vi "Excel Driver.vi"(0 "Filename of Workbook":path, 2 "Operator":T1, 5 "WorkSheet Name":string="Sheet 1", 7 "Range String\n(Or Search String)":string, 9 "Cell Values INPUT":string[][](array[string]), 11 "error in (no error)":errorcluster) -> (4 "Cell Values OUT":string[][](array[string]), 6 "Returned Range":string[](array[string]), 15 "error out":errorcluster)   [LabVIEW 2019]
uses:
  Type Defs/Excel Driver Operator Type Def.ctl
panel:
  in  "Excel._Worksheet Typecast Reference":refnum<k7>
  in  "Excel._Application Starter Reference":refnum<k7>
  # "C:\\My Documents\\MyLabviewFiles\\MDMachines\\Machine list 12-02-2002a.xls"
  # "Machine List"
  # "\\\\Dlbm32221\\MachineFolders\\Machine list 12-02-2002a.xls"
  # "C:\\Documents and Settings\\tz92qf\\My Documents\\MyLabview\\MDMachines\\Machine list 12-02-2002a.xls"
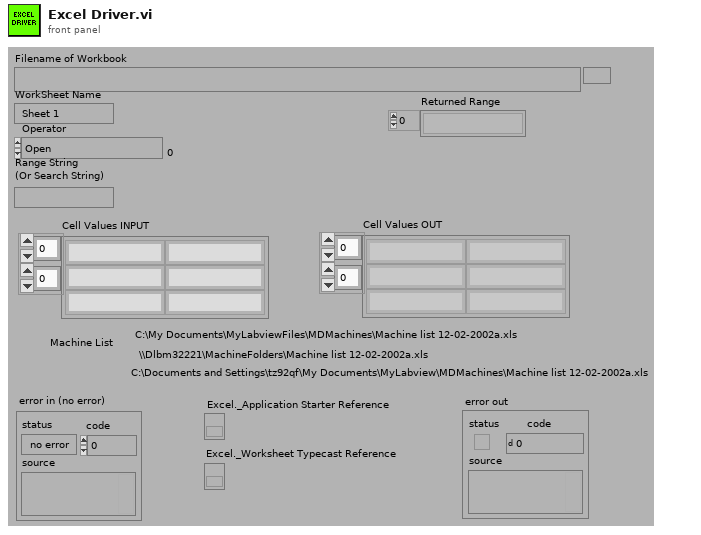
[diagram p1: front panel]
types:
  T1 = typedef "Excel Driver Operator Type Def.ctl" = enum16{"Open", "Close", "Search for String", "GetUsedRange", "Read Range", "Read Cell", "Set Range", "Set Cell"}
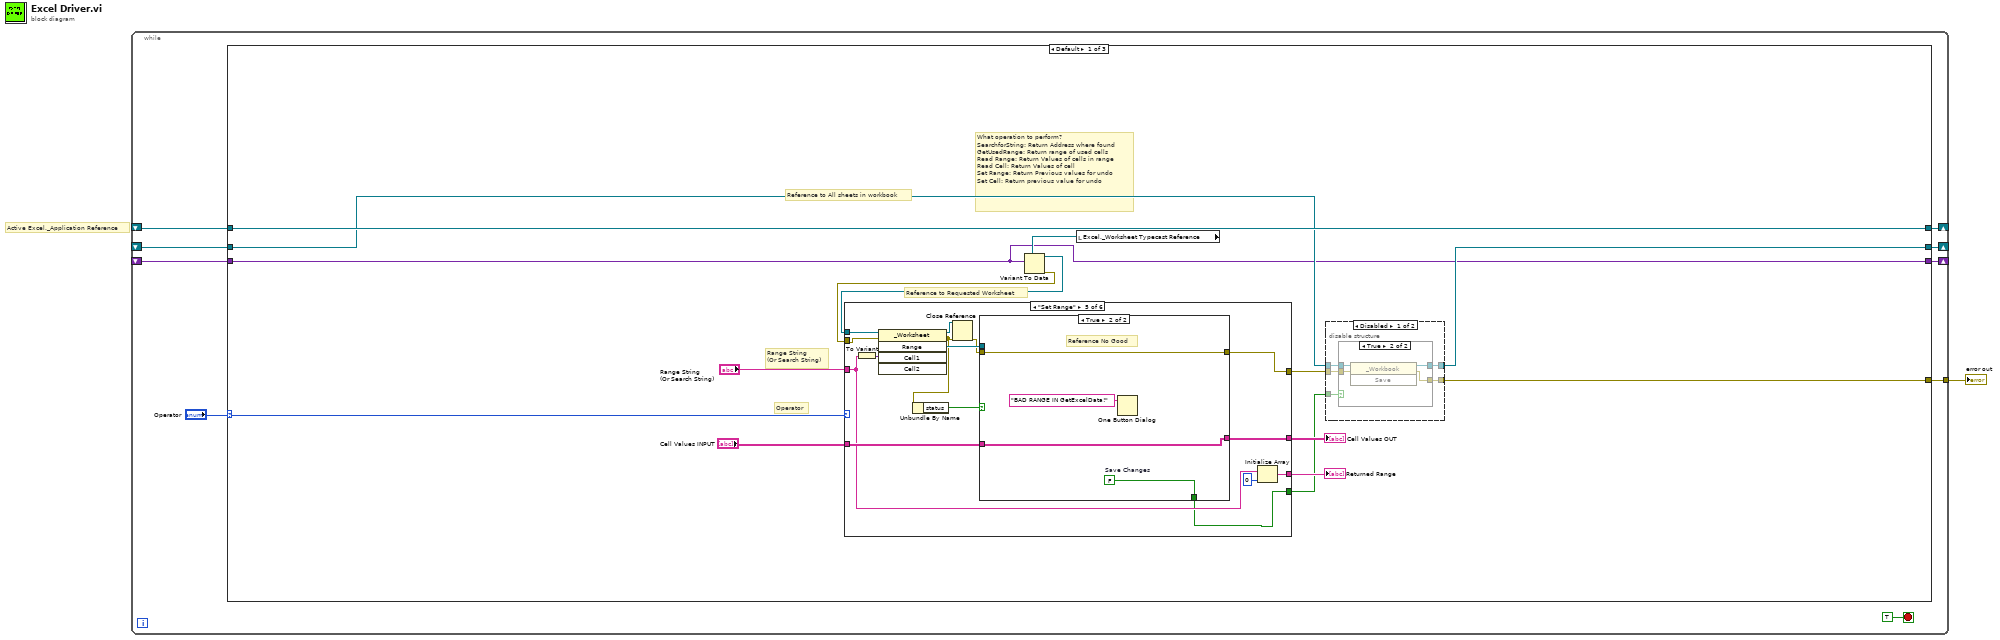
[diagram p0: block diagram]
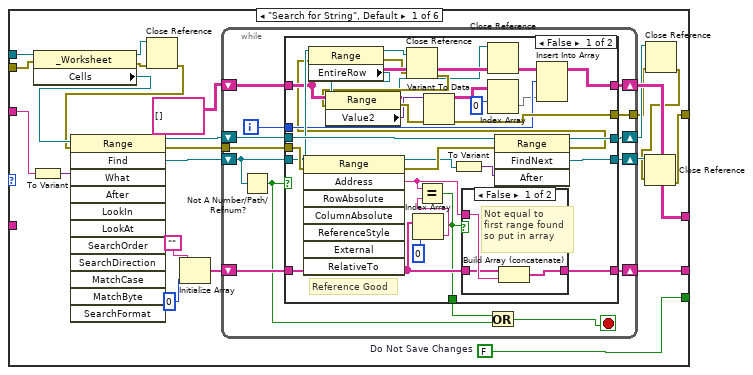
[diagram p4: hidden frame]
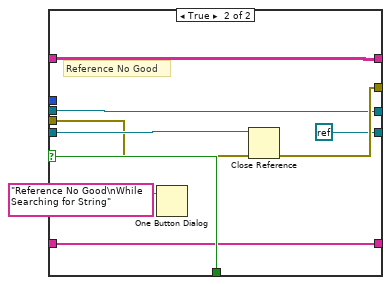
[diagram p6: hidden frame]
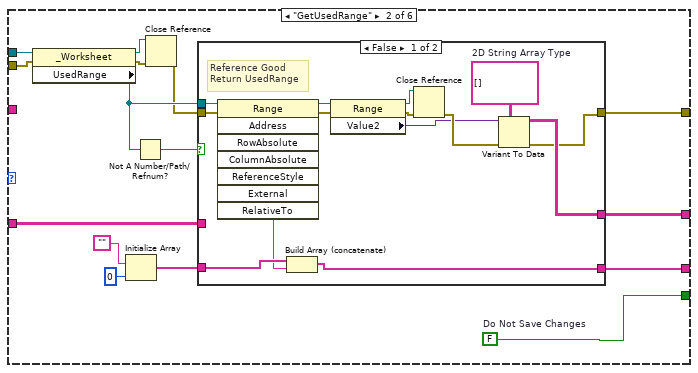
[diagram p7: hidden frame]
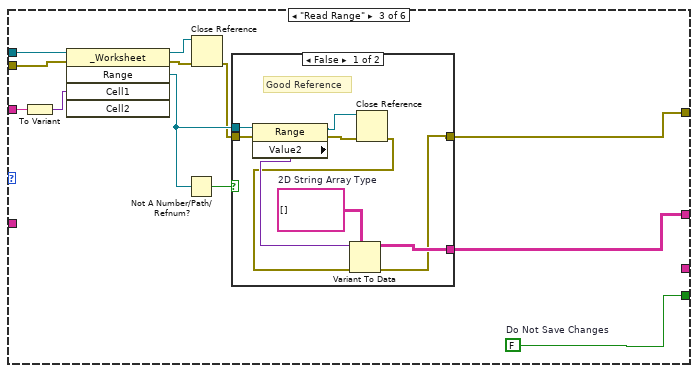
[diagram p9: hidden frame]
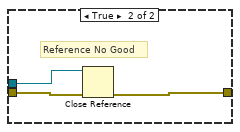
[diagram p10: hidden frame]
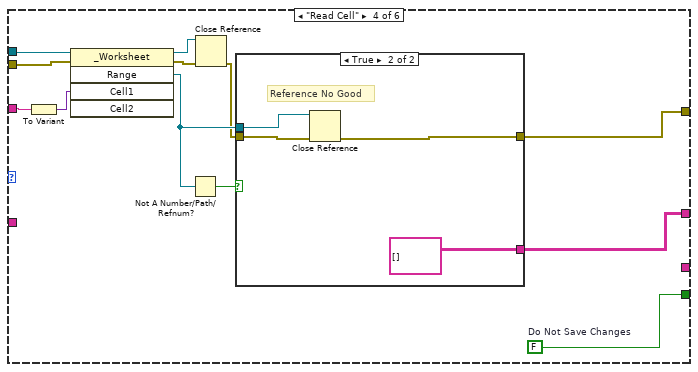
[diagram p11: hidden frame]
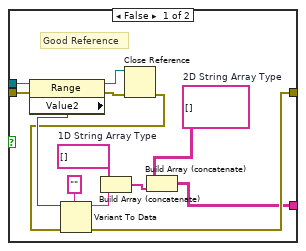
[diagram p12: hidden frame]
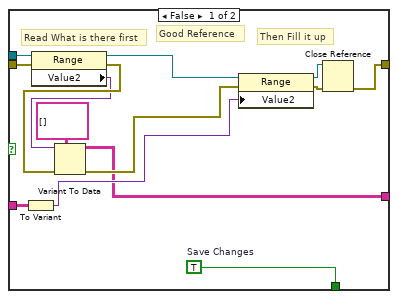
[diagram p13: hidden frame]
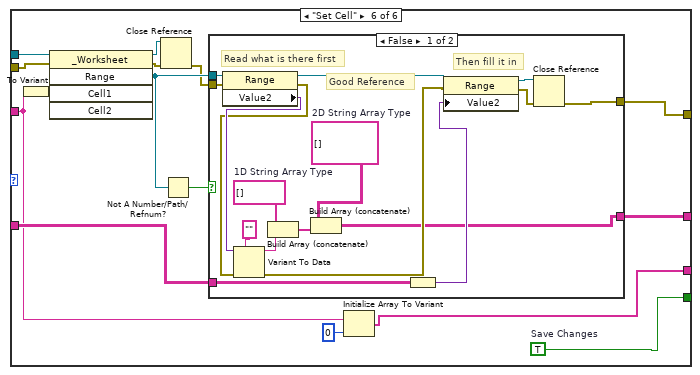
[diagram p14: hidden frame]
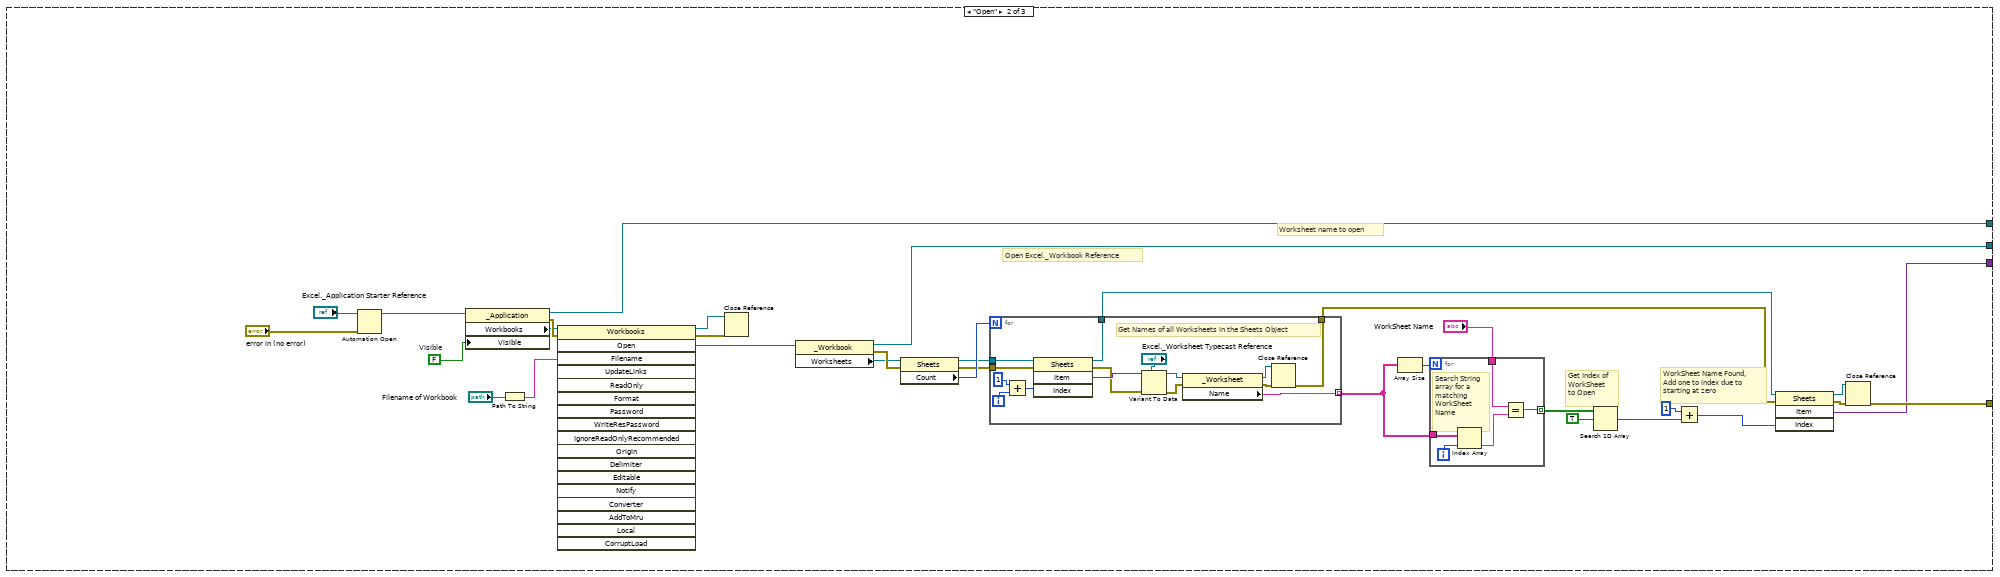
[diagram p16: hidden frame]
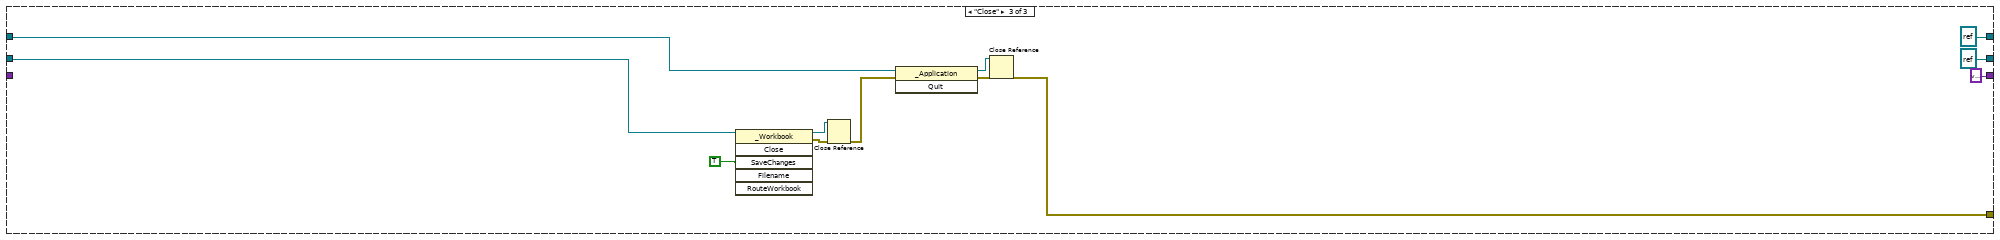
[diagram p17: hidden frame]
diagram:
  # "Active Excel._Application Reference"
  n1 = while {
    shift-right: [w10] -> _
    shift-left: _ -> [w9]
    tunnel: [w4] -> w1
    shift-right: [w6] -> _
    shift-left: _ -> [w5]
    shift-right: [w3] -> _
    shift-left: _ -> [w2]
    stop <- TRUE stop-if-true
    n2 = case shown="Default" "Operator" {
      selector: "Operator" -> [w24 _ _]
      tunnel: [w15 w280 refnum<k7> refnum ("Open")] -> w10
      tunnel: w9 -> [w16 _ w326]
      tunnel: [w19 w279 refnum<k7> refnum ("Excel._Application Starter Reference")] -> w6
      tunnel: w5 -> [w19 _ w327]
      tunnel: [w18 w271 w331] -> w4
      tunnel: [w11 w270 variant ("Item")] -> w3
      tunnel: w2 -> [w11 _ _]
      frame Default {
        # "Reference to Requested Worksheet"
        # "Range String\n(Or Search String)"
        # "Operator"
        # "Reference to All sheets in workbook"
        # "What operation to perform?\nSearchforString: Return Address where found\nGetUsedRange: Return range of used cells\nRead Range: Return Values of cells in range\nRead Cell: Return Values of cell\nSet Range: Return Previous values for undo\nSet Cell: Return previous value for undo"
        n3 = local read "Excel._Worksheet Typecast Reference"() -> (w12:refnum<k7>)
        n4 = Variant To Data(type=w12, Variant=w11) -> (data=w14:refnum<k7>, error out=w13:errorcluster)  [unwired: 1 in]
        n5 = case shown="\"Set Range\"" w24 {
          tunnel: w14 -> [w61 w130 w160 w177 w217 w245]
          tunnel: w13 -> [w60 w129 w161 w176 w216 w244]
          tunnel: "Range String\n(Or Search String)" -> [w59 _ w151 w175 w204 w239]
          tunnel: [w44 w126 w153 w178 w214 w241] -> w22
          tunnel: [w39 w118 w150 w174 w203 w236] -> w17
          tunnel: [w51 w122 _ _ w212 w237] -> w20
          tunnel: [w46 w120 w152 w179 w215 w240] -> w21
          tunnel: "Cell Values INPUT" -> [_ w119 _ _ w205 w242]
          frame "Search for String", Default {
            w39 = FALSE  # Do Not Save Changes
            n6 = To Variant(anything=w59) -> (Variant=w55:variant)
            n7 = property class="_Worksheet"(reference=w61, error in=w60) -> (reference out=w58:refnum<k7>, error out=w57:errorcluster, "Cells"=w56:refnum<k7>)
            n8 = Close Reference(reference=w58, error in (no error)=w57) -> (error out=w54:errorcluster)
            n9 = invoke class="Range" method="Find"(reference=w56, error in=w54, "What"=w55) -> (reference out=w43:refnum<k7>, error out=w52:errorcluster, "Find"=w53:refnum<k7>)  [unwired: 9 in, 9 out]
            n10 = Initialize Array("", 0 ("dimension size")) -> (w48:string[])
            n11 = while {
              shift-right: [w70] -> w51
              shift-left: w48 -> [w71]
              shift-right: [w73] -> w45
              shift-left: w53 -> [w75]
              tunnel: w52 -> [w74]
              tunnel: [w72] -> w41
              shift-right: [w64] -> w46
              shift-left: string[][] [] -> [w65]
              shift-right: [w63] -> w42
              shift-left: w43 -> [w62]
              i -> [w66]
              stop <- w67 stop-if-true
              n12 = Not A Number/Path/Refnum?(number/path/refnum=w75) -> (NaN/Path/Refnum?=w68:bool)
              n13 = case shown="False" w68 {
                selector: w68 -> [_ w117]
                tunnel: w75 -> [w92 w114]
                tunnel: w74 -> [w104 w110]
                tunnel: w62 -> [w103 w111]
                tunnel: [w101 refnum<k0> refnum] -> w73
                tunnel: [w90 w113] -> w72
                tunnel: w71 -> [w98 w116]
                tunnel: [w97 w116] -> w70
                tunnel: [w96 w117] -> w69
                tunnel: w66 -> [w85 _]
                tunnel: w65 -> [w83 w115]
                tunnel: [w82 w115] -> w64
                tunnel: [w77 w111] -> w63
                frame False {
                  # "Reference Good"
                  n14 = invoke class="Range" method="Address"(reference=w92, error in=w104) -> (reference out=w93:refnum<k7>, error out=w102:errorcluster, "Address"=w94:string)  [unwired: 6 in, 5 out]
                  n15 = Index Array(array=w98, index=0) -> (element=w99:string)
                  n16 = Equal?(x=w94, y=w99) -> (x = y?=w96:bool)
                  n17 = To Variant(anything=w93) -> (Variant=w95:variant)
                  n18 = case shown="False" w96 {
                    tunnel: w94 -> [w107 _]
                    tunnel: w98 -> [w106 w108]
                    tunnel: [w105 w108] -> w97
                    frame False {
                      # "Not equal to\nfirst range found\nso put in array"
                      n19 = Build Array (concatenate)(w106, w107) -> (w105:string[])
                    }
                    frame True {
                      # "Equal to\nfirst range found\nso that's all"
                    }
                  }
                  n20 = invoke class="Range" method="FindNext"(reference=w103, error in=w102, "After"=w95) -> (reference out=w77:refnum<k7>, error out=w76:errorcluster, "FindNext"=w101:refnum<k7>)  [unwired: 1 in, 1 out]
                  n21 = property class="Range"(reference=w92, error in=w76) -> (reference out=w81:refnum<k7>, error out=w80:errorcluster, "EntireRow"=w89:refnum<k7>)
                  n22 = Close Reference(reference=w81, error in (no error)=w80) -> (error out=w79:errorcluster)
                  n23 = property class="Range"(reference=w89, error in=w79) -> (reference out=w78:refnum<k7>, error out=w91:errorcluster, "Value2"=w88:variant)
                  n24 = Variant To Data(error in=w91, type=w83, Variant=w88) -> (data=w87:string[][], error out=w90:errorcluster)
                  n25 = Close Reference(reference=w78) -> ()  [unwired: 1 in, 1 out]
                  n26 = Index Array(array=w87, index (row)=0) -> (element=w84:string[])  [unwired: 1 in]
                  n27 = Insert Into Array(array=w83, index (row)=w85, new element=w84) -> (w82:string[][])  [unwired: 1 in]
                }
                frame True {
                  # "Reference No Good"
                  n28 = One Button Dialog(message="Reference No Good\nWhile Searching for String") -> ()  [unwired: 1 in, 1 out]
                  n29 = Close Reference(reference=w114, error in (no error)=w110) -> (error out=w113:errorcluster)
                }
              }
              n30 = Or(x=w69, y=w68) -> (x .or. y?=w67:bool)
            }
            n31 = Close Reference(reference=w42, error in (no error)=w41) -> (error out=w40:errorcluster)
            n32 = Close Reference(reference=w45, error in (no error)=w40) -> (error out=w44:errorcluster)
          }
          frame "GetUsedRange" {
            w118 = FALSE  # Do Not Save Changes
            n33 = property class="_Worksheet"(reference=w130, error in=w129) -> (reference out=w132:refnum<k7>, error out=w131:errorcluster, "UsedRange"=w128:refnum<k7>)
            n34 = Initialize Array("", 0 ("dimension size")) -> (w123:string[])
            n35 = Not A Number/Path/Refnum?(number/path/refnum=w128) -> (NaN/Path/Refnum?=w127:bool)
            n36 = Close Reference(reference=w132, error in (no error)=w131) -> (error out=w121:errorcluster)
            n37 = case shown="False" w127 {
              tunnel: w128 -> [w146 _]
              tunnel: w121 -> [w145 w148]
              tunnel: [w133 w148] -> w126
              tunnel: w123 -> [w144 w149]
              tunnel: [w142 w149] -> w122
              tunnel: [w134 w147] -> w120
              tunnel: w119 -> [_ w147]
              frame False {
                w138 = string[][] []  # 2D String Array Type
                # "Reference Good\nReturn UsedRange"
                n38 = invoke class="Range" method="Address"(reference=w146, error in=w145) -> (reference out=w141:refnum<k7>, error out=w140:errorcluster, "Address"=w143:string)  [unwired: 6 in, 5 out]
                n39 = Build Array (concatenate)(w144, w143) -> (w142:string[])
                n40 = property class="Range"(reference=w141, error in=w140) -> (reference out=w139:refnum<k7>, error out=w137:errorcluster, "Value2"=w135:variant)
                n41 = Close Reference(reference=w139, error in (no error)=w137) -> (error out=w136:errorcluster)
                n42 = Variant To Data(error in=w136, type=w138, Variant=w135) -> (data=w134:string[][], error out=w133:errorcluster)
              }
              frame True {
                # "Reference No Good,\nNo Used Range"
              }
            }
          }
          frame "Read Range" {
            w150 = FALSE  # Do Not Save Changes
            n43 = To Variant(anything=w151) -> (Variant=w159:variant)
            n44 = invoke class="_Worksheet" method="Range"(reference=w160, error in=w161, "Cell1"=w159) -> (reference out=w156:refnum<k7>, error out=w157:errorcluster, "Range"=w155:refnum<k7>)  [unwired: 2 in, 2 out]
            n45 = Not A Number/Path/Refnum?(number/path/refnum=w155) -> (NaN/Path/Refnum?=w158:bool)
            n46 = Close Reference(reference=w156, error in (no error)=w157) -> (error out=w154:errorcluster)
            n47 = case shown="False" w158 {
              tunnel: w155 -> [w170 w173]
              tunnel: w154 -> [w169 w172]
              tunnel: [w165 w171] -> w153
              tunnel: [w166 _] -> w152
              frame False {
                w167 = string[][] []  # 2D String Array Type
                # "Good Reference"
                n48 = property class="Range"(reference=w170, error in=w169) -> (reference out=w162:refnum<k7>, error out=w163:errorcluster, "Value2"=w168:variant)
                n49 = Close Reference(reference=w162, error in (no error)=w163) -> (error out=w164:errorcluster)
                n50 = Variant To Data(error in=w164, type=w167, Variant=w168) -> (data=w166:string[][], error out=w165:errorcluster)
              }
              frame True {
                # "Reference No Good"
                n51 = Close Reference(reference=w173, error in (no error)=w172) -> (error out=w171:errorcluster)
              }
            }
          }
          frame "Read Cell" {
            w174 = FALSE  # Do Not Save Changes
            n52 = To Variant(anything=w175) -> (Variant=w185:variant)
            n53 = invoke class="_Worksheet" method="Range"(reference=w177, error in=w176, "Cell1"=w185) -> (reference out=w182:refnum<k7>, error out=w183:errorcluster, "Range"=w181:refnum<k7>)  [unwired: 2 in, 2 out]
            n54 = Not A Number/Path/Refnum?(number/path/refnum=w181) -> (NaN/Path/Refnum?=w184:bool)
            n55 = Close Reference(reference=w182, error in (no error)=w183) -> (error out=w180:errorcluster)
            n56 = case shown="True" w184 {
              tunnel: w181 -> [w198 w202]
              tunnel: w180 -> [w197 w201]
              tunnel: [w195 w200] -> w178
              tunnel: [w193 string[][] [] ("2D String Array Type")] -> w179
              frame False {
                w191 = string[] []  # 1D String Array Type
                w194 = string[][] []  # 2D String Array Type
                # "Good Reference"
                n57 = property class="Range"(reference=w198, error in=w197) -> (reference out=w188:refnum<k7>, error out=w187:errorcluster, "Value2"=w196:variant)
                n58 = Close Reference(reference=w188, error in (no error)=w187) -> (error out=w186:errorcluster)
                n59 = Variant To Data(error in=w186, type="", Variant=w196) -> (data=w190:string, error out=w195:errorcluster)
                n60 = Build Array (concatenate)(w191, w190) -> (w189:string[])
                n61 = Build Array (concatenate)(w194, w189) -> (w193:string[][])
              }
              frame True {
                # "Reference No Good"
                n62 = Close Reference(reference=w202, error in (no error)=w201) -> (error out=w200:errorcluster)
              }
            }
          }
          frame "Set Range" {
            n63 = To Variant(anything=w204) -> (Variant=w211:variant)
            n64 = invoke class="_Worksheet" method="Range"(reference=w217, error in=w216, "Cell1"=w211) -> (reference out=w209:refnum<k7>, error out=w207:errorcluster, "Range"=w210:refnum<k7>)  [unwired: 2 in, 2 out]
            n65 = Unbundle By Name(w207) -> ("status"=w206:bool)
            n66 = Close Reference(reference=w209, error in (no error)=w207) -> (error out=w208:errorcluster)
            n67 = case shown="True" w206 {
              tunnel: w208 -> [w228 w234]
              tunnel: w205 -> [w224 w235]
              tunnel: [w218 w235] -> w215
              tunnel: [w231 w234] -> w214
              tunnel: w210 -> [w229 _]
              tunnel: [w221 w233] -> w203
              frame False {
                w221 = TRUE  # Save Changes
                # "Then Fill it up"
                # "Read What is there first"
                # "Good Reference"
                n68 = To Variant(anything=w224) -> (Variant=w220:variant)
                n69 = property class="Range"(reference=w229, error in=w228) -> (reference out=w230:refnum<k7>, error out=w226:errorcluster, "Value2"=w219:variant)
                n70 = Variant To Data(error in=w226, type=string[][] [], Variant=w219) -> (data=w218:string[][], error out=w227:errorcluster)
                n71 = property class="Range"(reference=w230, error in=w227, "Value2"=w220) -> (reference out=w223:refnum<k7>, error out=w222:errorcluster)
                n72 = Close Reference(reference=w223, error in (no error)=w222) -> (error out=w231:errorcluster)
              }
              frame True {
                w233 = FALSE  # Save Changes
                # "Reference No Good"
                n73 = One Button Dialog(message="BAD RANGE IN GetExcelData!") -> ()  [unwired: 1 in, 1 out]
              }
            }
            n74 = Initialize Array(w204, 0 ("dimension size")) -> (w212:string[])
          }
          frame "Set Cell" {
            w236 = TRUE  # Save Changes
            n75 = To Variant(anything=w239) -> (Variant=w250:variant)
            n76 = invoke class="_Worksheet" method="Range"(reference=w245, error in=w244, "Cell1"=w250) -> (reference out=w248:refnum<k7>, error out=w249:errorcluster, "Range"=w247:refnum<k7>)  [unwired: 2 in, 2 out]
            n77 = Close Reference(reference=w248, error in (no error)=w249) -> (error out=w246:errorcluster)
            n78 = Not A Number/Path/Refnum?(number/path/refnum=w247) -> (NaN/Path/Refnum?=w243:bool)
            n79 = case shown="False" w243 {
              tunnel: w247 -> [w267 _]
              tunnel: w246 -> [w266 w269]
              tunnel: w242 -> [w253 w268]
              tunnel: [w252 w269] -> w241
              tunnel: [w251 w268] -> w240
              frame False {
                w261 = string[] []  # 1D String Array Type
                w263 = string[][] []  # 2D String Array Type
                # "Read what is there first"
                # "Then fill it in"
                # "Good Reference"
                n80 = property class="Range"(reference=w267, error in=w266) -> (reference out=w255:refnum<k7>, error out=w264:errorcluster, "Value2"=w265:variant)
                n81 = Variant To Data(error in=w264, type="", Variant=w265) -> (data=w260:string, error out=w254:errorcluster)
                n82 = Build Array (concatenate)(w261, w260) -> (w259:string[])
                n83 = Build Array (concatenate)(w263, w259) -> (w251:string[][])
                n84 = To Variant(anything=w253) -> (Variant=w258:variant)
                n85 = property class="Range"(reference=w255, error in=w254, "Value2"=w258) -> (reference out=w256:refnum<k7>, error out=w257:errorcluster)
                n86 = Close Reference(reference=w256, error in (no error)=w257) -> (error out=w252:errorcluster)
              }
              frame True {
                # "Reference No Good"
              }
            }
            n87 = Initialize Array(w239, 0 ("dimension size")) -> (w237:string[])
          }
        }
        "Returned Range" <- w20
        "Cell Values OUT" <- w21
        n88 = disable-structure shown="Disabled" {
          disable-tunnel: w22 -> [w30 w37]
          disable-tunnel: [w29 w37] -> w18
          disable-tunnel: w17 -> [w28 _]
          disable-tunnel: w16 -> [w27 w38]
          disable-tunnel: [w26 w38] -> w15
          frame Disabled {
            n89 = case shown="True" w28 {
              tunnel: w30 -> [w32 w36]
              tunnel: [w32 w35] -> w29
              tunnel: w27 -> [w31 w34]
              tunnel: [w31 w33] -> w26
              frame False {
              }
              frame True {
                n90 = invoke class="_Workbook" method="Save"(reference=w34, error in=w36) -> (reference out=w33:refnum<k7>, error out=w35:errorcluster)  [unwired: 1 in, 1 out]
              }
            }
          }
          frame Enabled {
          }
        }
      }
      frame "Open" {
        w292 = FALSE  # Visible
        # "WorkSheet Name Found,\nAdd one to index due to\nstarting at zero"
        # "Get Index of\nWorkSheet\nto Open"
        # "Open Excel._Workbook Reference"
        # "Worksheet name to open"
        n91 = Automation Open(error in (no error)="error in (no error)", Automation Refnum="Excel._Application Starter Reference") -> (Automation Refnum=w287:refnum<k7>)  [unwired: 2 in, 1 out]
        n92 = property class="_Application"(reference=w287, "Visible"=w292) -> (reference out=w279:refnum<k7>, error out=w293:errorcluster, "Workbooks"=w291:refnum<k7>)  [unwired: 1 in]
        n93 = Path To String(path="Filename of Workbook") -> (string=w294:string)
        n94 = invoke class="Workbooks" method="Open"(reference=w291, error in=w293, "Filename"=w294) -> (reference out=w290:refnum<k7>, error out=w289:errorcluster, "Open"=w288:refnum<k7>)  [unwired: 15 in, 15 out]
        n95 = Close Reference(reference=w290, error in (no error)=w289) -> ()  [unwired: 1 out]
        n96 = property class="_Workbook"(reference=w288) -> (reference out=w280:refnum<k7>, error out=w296:errorcluster, "Worksheets"=w295:refnum<k7>)  [unwired: 1 in]
        n97 = property class="Sheets"(reference=w295, error in=w296) -> (reference out=w297:refnum<k7>, error out=w298:errorcluster, "Count"=w299:i32)
        n98 = for {
          N: w299 -> [_]
          tunnel: w297 -> [w321]
          tunnel: w298 -> [w318]
          tunnel: [w311] -> w282 mode=indexing
          tunnel: [w308] -> w273
          tunnel: [w307] -> w272
          i -> [w316]
          # "Get Names of all Worksheets in the Sheets Object"
          n99 = Add(x=1, y=w316) -> (x+y=w314:i32)
          n100 = invoke class="Sheets" method="Item"(reference=w321, error in=w318, "Index"=w314) -> (reference out=w308:refnum<k7>, error out=w310:errorcluster, "Item"=w320:variant)  [unwired: 1 in, 1 out]
          n101 = Variant To Data(error in=w310, type="Excel._Worksheet Typecast Reference", Variant=w320) -> (data=w309:refnum<k7>, error out=w317:errorcluster)
          n102 = property class="_Worksheet"(reference=w309, error in=w317) -> (reference out=w312:refnum<k7>, error out=w313:errorcluster, "Name"=w311:string)
          n103 = Close Reference(reference=w312, error in (no error)=w313) -> (error out=w307:errorcluster)
        }
        n104 = Array Size(array=w282) -> (size(s)=w285:i32)
        n105 = for {
          N: w285 -> [_]
          tunnel: w282 -> [w306]
          tunnel: [w305] -> w283 mode=indexing
          tunnel: "WorkSheet Name" -> [w302]
          i -> [w303]
          # "Search String\narray for a\nmatching\nWorkSheet\nName"
          n106 = Index Array(array=w306, index=w303) -> (element=w304:string)
          n107 = Equal?(x=w302, y=w304) -> (x = y?=w305:bool)
        }
        n108 = Search 1D Array(1D array=w283, element=TRUE) -> (index of element=w274:i32)  [unwired: 1 in]
        n109 = Add(x=1 ("y"), y=w274) -> (x+y=w278:i32)
        n110 = invoke class="Sheets" method="Item"(reference=w273, error in=w272, "Index"=w278) -> (reference out=w276:refnum<k7>, error out=w275:errorcluster, "Item"=w270:variant)  [unwired: 1 in, 1 out]
        n111 = Close Reference(reference=w276, error in (no error)=w275) -> (error out=w271:errorcluster)
      }
      frame "Close" {
        n112 = invoke class="_Workbook" method="Close"(reference=w326, "SaveChanges"=TRUE) -> (reference out=w330:refnum<k7>, error out=w329:errorcluster)  [unwired: 4 in, 4 out]
        n113 = Close Reference(reference=w330, error in (no error)=w329) -> (error out=w325:errorcluster)
        n114 = invoke class="_Application" method="Quit"(reference=w327, error in=w325) -> (reference out=w332:refnum<k7>, error out=w333:errorcluster)  [unwired: 1 in, 1 out]
        n115 = Close Reference(reference=w332, error in (no error)=w333) -> (error out=w331:errorcluster)
      }
    }
  }
  "error out" <- w1
